vi "Get Random Ephemeral TCP Port.vi"() -> (3 "ephemeral TCP port":u16)   [LabVIEW 2013]
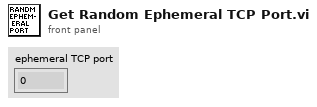
[diagram p1: front panel]
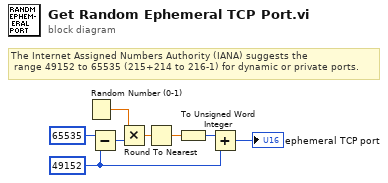
[diagram p0: block diagram]
diagram:
  w3 = u16 49152 ("x")
  # "The Internet Assigned Numbers Authority (IANA) suggests the\n range 49152 to 65535 (215+214 to 216-1) for dynamic or private ports."
  n1 = Random Number (0-1)() -> (number: 0 to 1=w6:dbl)
  n2 = Subtract(x=u16 65535, y=w3) -> (x-y=w7:u16)
  n3 = Multiply(x=w6, y=w7) -> (x*y=w5:dbl)
  n4 = Round To Nearest(number=w5) -> (nearest integer value=w4:dbl)
  n5 = To Unsigned Word Integer(number=w4) -> (unsigned 16bit integer=w2:u16)
  n6 = Add(x=w2, y=w3) -> (x+y=→"ephemeral TCP port":u16)
